vi "Destroy Promise.vi"(8 "error in (no error)":errorcluster, 11 "Promise in":refnum<class "Promise.lvclass">) -> (0 "error out":errorcluster)   [LabVIEW 2017, in "Promise.lvlib" / "Promise.lvclass"]
doc: "Destroys the Promise, causing any Read or Write attempts to error immediately."
uses:
  Promise.lvclass
  Promise.lvclass/Promise.ctl
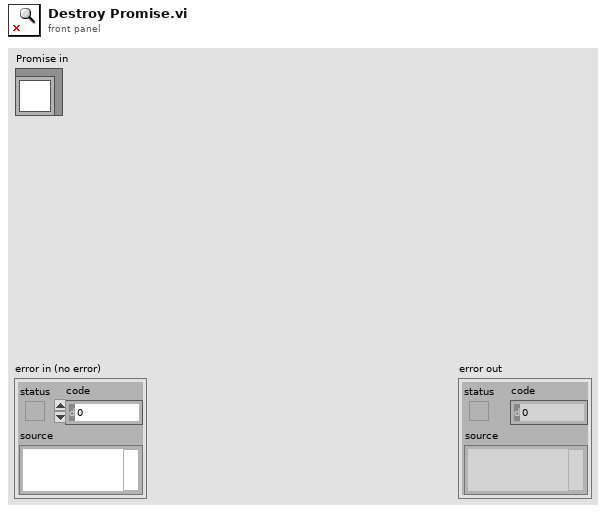
[diagram p1: front panel]
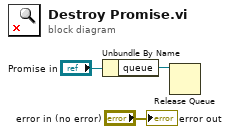
[diagram p0: block diagram]
diagram:
  n1 = Unbundle By Name("Promise in") -> ("queue"=w1:refnum<queue>)
  n2 = Release Queue(queue=w1) -> ()  [unwired: 2 in, 3 out]
  "error out" <- "error in (no error)"
